vi "U6 Quadrature 2-Input Configure.vi"(8 "error in":errorcluster, 11 "Handle In":i32) -> (0 "error out":errorcluster, 3 "Handle Out":i32)   [LabVIEW 2021]
panel:
  out "Error Message":string
  # "Configures 2 quadrature inputs.  The first uses Timer0/Timer1 on FIO0/FIO1 for phases A & B.  The\nsecond uses Timer2/Timer3 on FIO2/FIO3 for phases A & B."
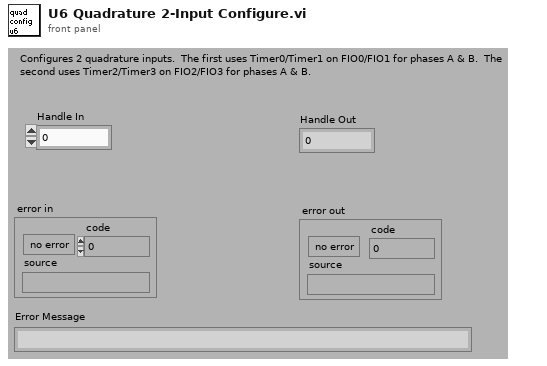
[diagram p1: front panel]
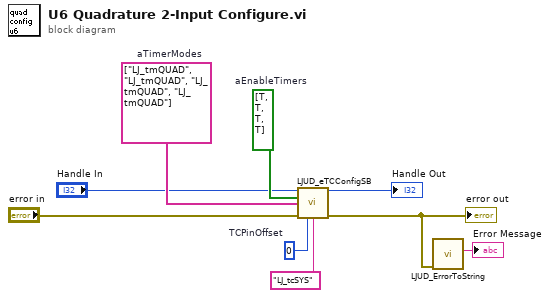
[diagram p0: block diagram]
diagram:
  w6 = 0  # TCPinOffset
  w5 = bool[] [TRUE, TRUE, TRUE, TRUE]  # aEnableTimers
  w8 = string[] ["LJ_tmQUAD", "LJ_tmQUAD", "LJ_tmQUAD", "LJ_tmQUAD"]  # aTimerModes
  n1 = call "LJUD_eTCConfigSB.vi"("Handle In"="Handle In", "aEnableTimers"=w5, "aTimerModes"=w8, "error in"="error in", "TCPinOffset"=w6, "TimerClockBase"="LJ_tcSYS") -> ("Handle Out"=→"Handle Out":i32, "error out"=w4:errorcluster)  [unwired: 8 in]
  "error out" <- w4
  n2 = call "LJUD_ErrorToString.vi"("error in"=w4) -> ("String"=→"Error Message":string)  [unwired: 10 in]
